vi "Launcher.vi"() -> ()   [LabVIEW 2020]
uses:
  <vilib>/ActorFramework/Message Enqueuer/Message Enqueuer.lvclass
  <vilib>/ActorFramework/Message Enqueuer/Message Enqueuer.lvclass/Message Enqueuer.ctl
  C:/Program Files (x86)/National Instruments/LabVIEW 2020/vi.lib/ActorFramework/Actor/Actor.lvclass
  GUI DigitalCount/GUI DigitalCount.lvclass
  <vilib>/ActorFramework/Message Enqueuer/Enqueue.vi
  <vilib>/ActorFramework/Stop Msg/Stop Msg.lvclass
  C:/Program Files (x86)/National Instruments/LabVIEW 2020/vi.lib/ActorFramework/Message/Message.lvclass
  <vilib>/ActorFramework/Message Priority Queue/Priority Enqueue.vi
  <vilib>/ActorFramework/Actor/Actor.lvclass
panel:
  in  "Stop Button":bool
  in  "Cerrar Contador":bool
  in  "Cerrar Generador":bool
  in  "Contadores Abiertos":u16(ring)
  in  "Generadores Abiertos":u16(ring)
  in  "Contador Digital":bool
  in  "Generador De Funciones":bool
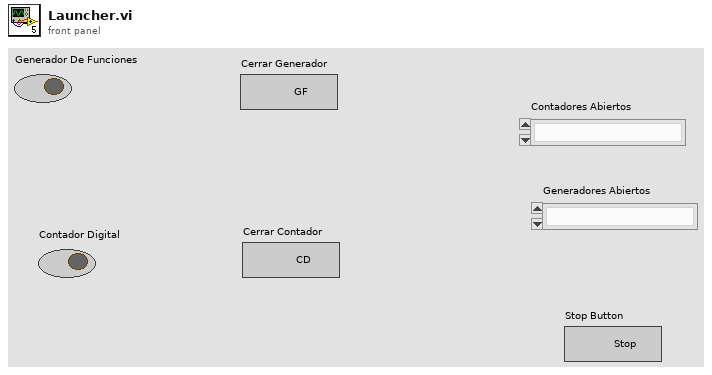
[diagram p1: front panel]
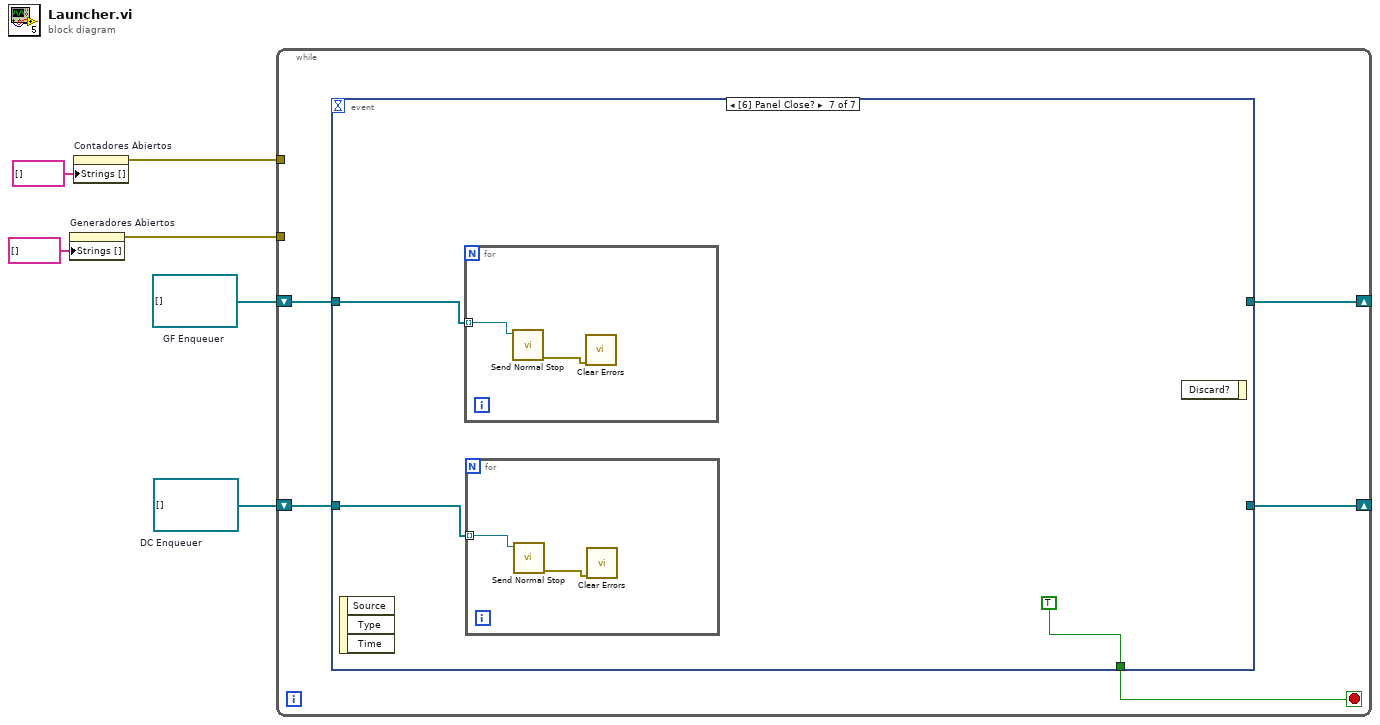
[diagram p0: block diagram]
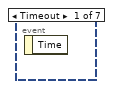
[diagram p2: hidden frame]
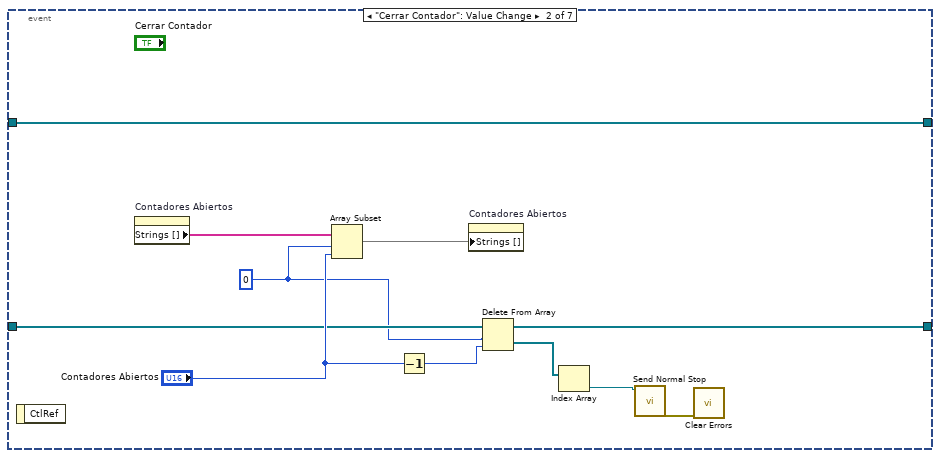
[diagram p3: hidden frame]
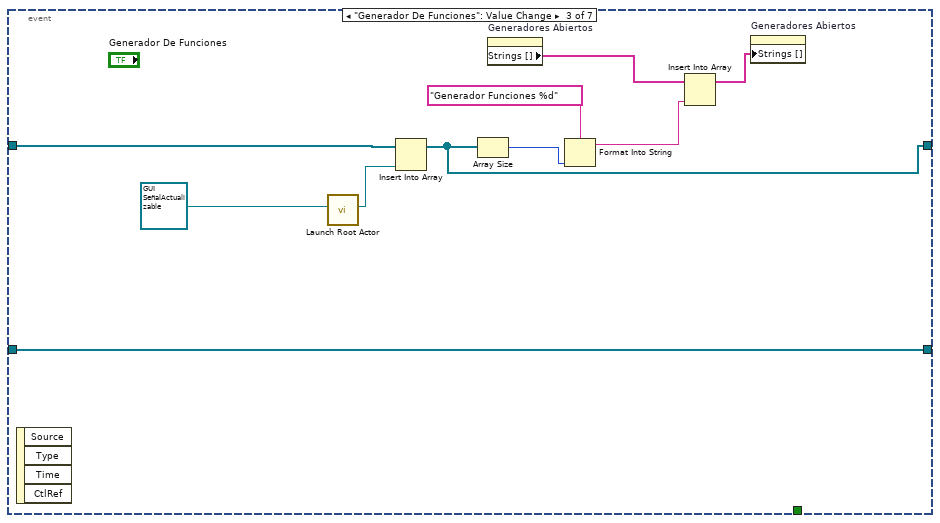
[diagram p4: hidden frame]
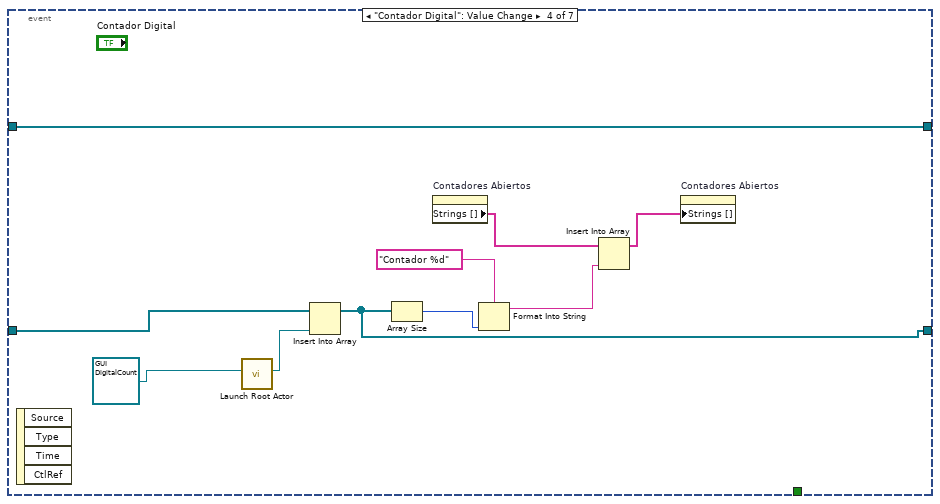
[diagram p5: hidden frame]
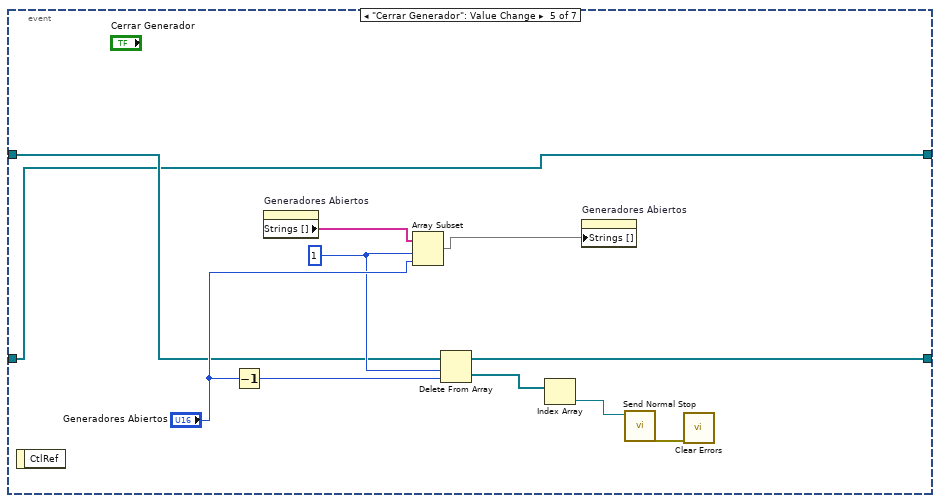
[diagram p6: hidden frame]
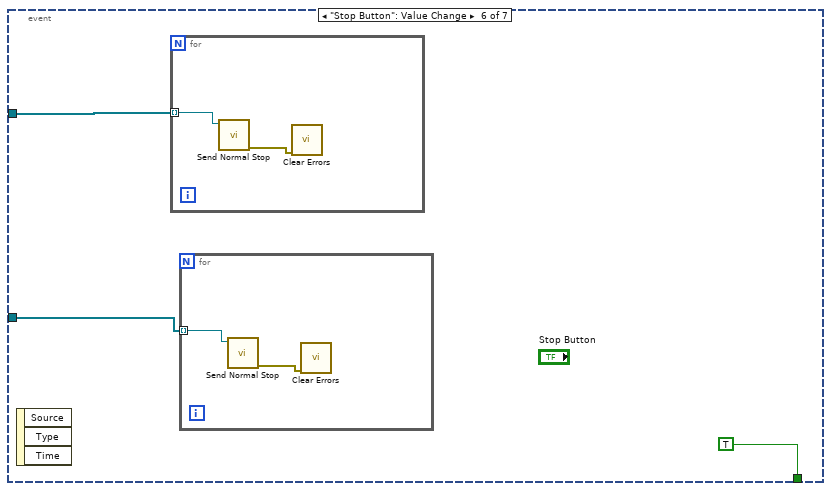
[diagram p7: hidden frame]
diagram:
  w1 = refnum<class "Message Enqueuer.lvclass">[] []  # DC Enqueuer
  w2 = refnum<class "Message Enqueuer.lvclass">[] []  # GF Enqueuer
  n1 = property on="Generadores Abiertos" class="Ring (strict)"("Strings []"=string[] []) -> (error out=w3:errorcluster)  [unwired: 2 in, 1 out]
  n2 = property on="Contadores Abiertos" class="Ring (strict)"("Strings []"=string[] []) -> (error out=w4:errorcluster)  [unwired: 2 in, 1 out]
  n3 = while {
    tunnel: w4 -> [_]
    tunnel: w3 -> [_]
    shift-right: [w10] -> _
    shift-left: w2 -> [w11]
    shift-right: [w8] -> _
    shift-left: w1 -> [w9]
    stop <- w7 stop-if-true
    n4 = event shown="[6] Panel Close?" {
      selector: _ -> [_ _ _ _ _ _ _]
      dyn-events: _ -> [_ _ _ _ _ _ _]
      timeout: _ -> [_ _ _ _ _ _ _]
      tunnel: [_ w12 w27 w42 w43 _ _] -> w10
      tunnel: w11 -> [_ w12 w31 w42 w44 w56 w63]
      tunnel: [_ w17 w29 w35 w45 _ _] -> w8
      tunnel: w9 -> [_ w16 w29 w36 w43 w55 w62]
      tunnel: [_ _ _ _ _ TRUE ("Stop Button") TRUE ("Stop Button")] -> w7
      event Timeout {
        n5 = event-data() -> ()  [unwired: 1 in, 1 out]
      }
      event "Cerrar Contador": Value Change {
        w15 = 0
        n6 = event-data() -> ()  [unwired: 1 in, 1 out]
        n7 = property on="Contadores Abiertos" class="Ring (strict)"() -> ("Strings []"=w22:string[])  [unwired: 2 in, 2 out]
        n8 = Array Subset(array=w22, index=w15, length="Contadores Abiertos") -> (w21:string[])
        n9 = Decrement(x="Contadores Abiertos") -> (x-1=w14:u16)
        n10 = property on="Contadores Abiertos" class="Ring (strict)"("Strings []"=w21) -> ()  [unwired: 2 in, 2 out]
        n11 = Delete From Array(array=w16, length=w15, index=w14) -> (deleted portion=w13:refnum<class "Message Enqueuer.lvclass">[], array with subset deleted=w17:refnum<class "Message Enqueuer.lvclass">[])
        n12 = Index Array(array=w13) -> (element=w19:refnum<class "Message Enqueuer.lvclass">)  [unwired: 1 in]
        n13 = call <vilib>:"Send Normal Stop.vi"("Message Enqueuer"=w19) -> ("error out"=w18:errorcluster)  [unwired: 10 in]
        n14 = call <vilib>:"Clear Errors.vi"("error in (no error)"=w18) -> ()  [unwired: 5 in, 2 out]
      }
      event "Generador De Funciones": Value Change {
        n15 = event-data() -> ()  [unwired: 1 in, 4 out]
        n16 = call <vilib>:"Launch Root Actor.vi"("Actor"=refnum<class "GUI SeñalActualizable.lvclass"> refnum ("GUI SeñalActualizable.lvlib:GUI SeñalActualizable.lvclass")) -> ("Actor's Enqueuer"=w30:refnum<class "Message Enqueuer.lvclass">)  [unwired: 9 in, 1 out]
        n17 = Insert Into Array(array=w31, new element=w30) -> (w27:refnum<class "Message Enqueuer.lvclass">[])  [unwired: 1 in]
        n18 = Array Size(array=w27) -> (size(s)=w28:i32)
        n19 = property on="Generadores Abiertos" class="Ring (strict)"() -> ("Strings []"=w24:string[])  [unwired: 2 in, 2 out]
        n20 = Format Into String(format string="Generador Funciones %d", w28) -> (resulting string=w25:string)  [unwired: 2 in, 1 out]
        n21 = Insert Into Array(array=w24, new element=w25) -> (w23:string[])  [unwired: 1 in]
        n22 = property on="Generadores Abiertos" class="Ring (strict)"("Strings []"=w23) -> ()  [unwired: 2 in, 2 out]
      }
      event "Contador Digital": Value Change {
        n23 = event-data() -> ()  [unwired: 1 in, 4 out]
        n24 = call <vilib>:"Launch Root Actor.vi"("Actor"=refnum<class "GUI DigitalCount.lvclass"> refnum ("GUI DigitalCount.lvlib:GUI DigitalCount.lvclass")) -> ("Actor's Enqueuer"=w41:refnum<class "Message Enqueuer.lvclass">)  [unwired: 9 in, 1 out]
        n25 = Insert Into Array(array=w36, new element=w41) -> (w35:refnum<class "Message Enqueuer.lvclass">[])  [unwired: 1 in]
        n26 = Array Size(array=w35) -> (size(s)=w40:i32)
        n27 = property on="Contadores Abiertos" class="Ring (strict)"() -> ("Strings []"=w33:string[])  [unwired: 2 in, 2 out]
        n28 = Format Into String(format string="Contador %d", w40) -> (resulting string=w38:string)  [unwired: 2 in, 1 out]
        n29 = Insert Into Array(array=w33, new element=w38) -> (w34:string[])  [unwired: 1 in]
        n30 = property on="Contadores Abiertos" class="Ring (strict)"("Strings []"=w34) -> ()  [unwired: 2 in, 2 out]
      }
      event "Cerrar Generador": Value Change {
        w49 = 1 ("index")
        n31 = event-data() -> ()  [unwired: 1 in, 1 out]
        n32 = Decrement(x="Generadores Abiertos") -> (x-1=w50:u16)
        n33 = property on="Generadores Abiertos" class="Ring (strict)"() -> ("Strings []"=w53:string[])  [unwired: 2 in, 2 out]
        n34 = Array Subset(array=w53, index=w49, length="Generadores Abiertos") -> (w52:string[])
        n35 = Delete From Array(array=w44, length=w49, index=w50) -> (deleted portion=w48:refnum<class "Message Enqueuer.lvclass">[], array with subset deleted=w45:refnum<class "Message Enqueuer.lvclass">[])
        n36 = Index Array(array=w48) -> (element=w47:refnum<class "Message Enqueuer.lvclass">)  [unwired: 1 in]
        n37 = property on="Generadores Abiertos" class="Ring (strict)"("Strings []"=w52) -> ()  [unwired: 2 in, 2 out]
        n38 = call <vilib>:"Send Normal Stop.vi"("Message Enqueuer"=w47) -> ("error out"=w46:errorcluster)  [unwired: 10 in]
        n39 = call <vilib>:"Clear Errors.vi"("error in (no error)"=w46) -> ()  [unwired: 5 in, 2 out]
      }
      event "Stop Button": Value Change {
        n40 = event-data() -> ()  [unwired: 1 in, 3 out]
        n41 = for {
          tunnel: w56 -> [w59] mode=indexing
          n42 = call <vilib>:"Send Normal Stop.vi"("Message Enqueuer"=w59) -> ("error out"=w60:errorcluster)  [unwired: 10 in]
          n43 = call <vilib>:"Clear Errors.vi"("error in (no error)"=w60) -> ()  [unwired: 5 in, 2 out]
        }
        n44 = for {
          tunnel: w55 -> [w57] mode=indexing
          n45 = call <vilib>:"Send Normal Stop.vi"("Message Enqueuer"=w57) -> ("error out"=w58:errorcluster)  [unwired: 10 in]
          n46 = call <vilib>:"Clear Errors.vi"("error in (no error)"=w58) -> ()  [unwired: 5 in, 2 out]
        }
      }
      event Panel Close? {
        n47 = event-data() -> ()  [unwired: 1 in, 3 out]
        n48 = for {
          tunnel: w63 -> [w66] mode=indexing
          n49 = call <vilib>:"Send Normal Stop.vi"("Message Enqueuer"=w66) -> ("error out"=w67:errorcluster)  [unwired: 10 in]
          n50 = call <vilib>:"Clear Errors.vi"("error in (no error)"=w67) -> ()  [unwired: 5 in, 2 out]
        }
        n51 = for {
          tunnel: w62 -> [w64] mode=indexing
          n52 = call <vilib>:"Send Normal Stop.vi"("Message Enqueuer"=w64) -> ("error out"=w65:errorcluster)  [unwired: 10 in]
          n53 = call <vilib>:"Clear Errors.vi"("error in (no error)"=w65) -> ()  [unwired: 5 in, 2 out]
        }
        n54 = event-data() -> ()  [unwired: 2 in, 1 out]
      }
    }
  }
